vi "Session Request - Brose Session.vi"(0 "ID Request":string="18DA55F2", 1 "ID Response":string="18DAF255") -> (2 "Data String":string, 3 "ID String":string, 4 "Write":refnum<k21>, 5 "Read":refnum<k21>)   [LabVIEW 2022 SP3]
panel:
  out "error out":errorcluster
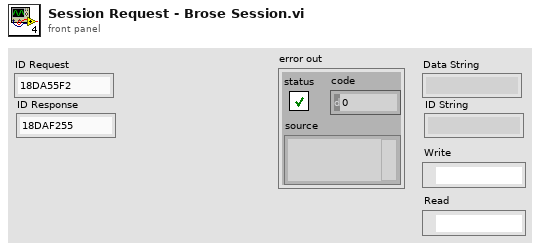
[diagram p1: front panel]
types:
  T1 = typedef "XNET Frame CAN.ctl" = cluster{"timestamp":timestamp, "payload":u8[], "identifier":u32, "type":T2, "extended?":bool, "echo?":bool}
  T2 = typedef "XNET Frame Type CAN.ctl" = u8
  T3 = cluster{"data[0]":T1, "data[1]":T1, "data[2]":T1, "data[3]":T1, "data[4]":T1, "data[5]":T1, "data[6]":T1, "data[7]":T1, "data[8]":T1}
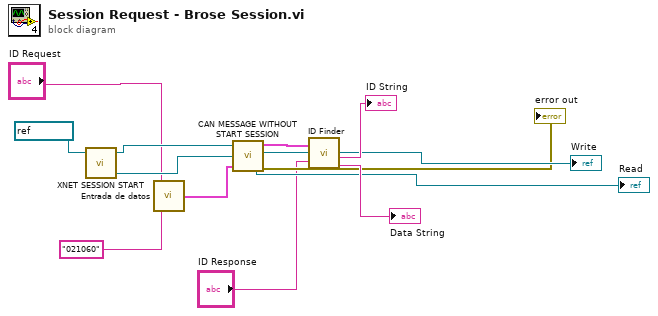
[diagram p0: block diagram]
diagram:
  n1 = call "XNET SESSION START.vi"("interface"=refnum<k21> "CAN1") -> ("Read"=w8:refnum<k21>, "Write"=w9:refnum<k21>)  [unwired: 2 in, 1 out]
  n2 = call "Entrada de datos.vi"("string"="021060", "ID"="ID Request") -> ("CAN frame"=w13:T1)
  n3 = call "CAN MESSAGE WITHOUT START SESSION.vi"("Write"=w9, "Read"=w8, "CAN frame"=w13) -> ("cluster"=w12:T3, "Write"=→"Write":refnum<k21>, "Read"=→"Read":refnum<k21>, "error out"=→"error out":errorcluster)
  n4 = call "ID Finder.vi"("cluster"=w12, "ID ESPERADO STRING"="ID Response") -> ("ID String"=→"ID String":string, "Data String"=→"Data String":string)  [unwired: 4 out]
